vi "Aula do dia 03.02.vi"() -> (0 "Corrente Fase A":dynamicdata(graph), 1 "Tensão Fase A":dynamicdata(graph), 2 "Timestamp":dynamicdata(graph), 3 "Corrente Fase C":dynamicdata(graph), 4 "Tensão Fase C":dynamicdata(graph), 5 "Corrente Fase B":dynamicdata(graph), 6 "Tensão Fase B":dynamicdata(graph))   [LabVIEW 2020]
panel:
  out "Fase C":string[][](table)
  out "Fase B":string[][](table)
  out "Fase A":string[][](table)
  out "Timestamp":string[][](table)
  out "Gráfico de Ondas":dynamicdata(graph)
  out "All Data":string[][](table)
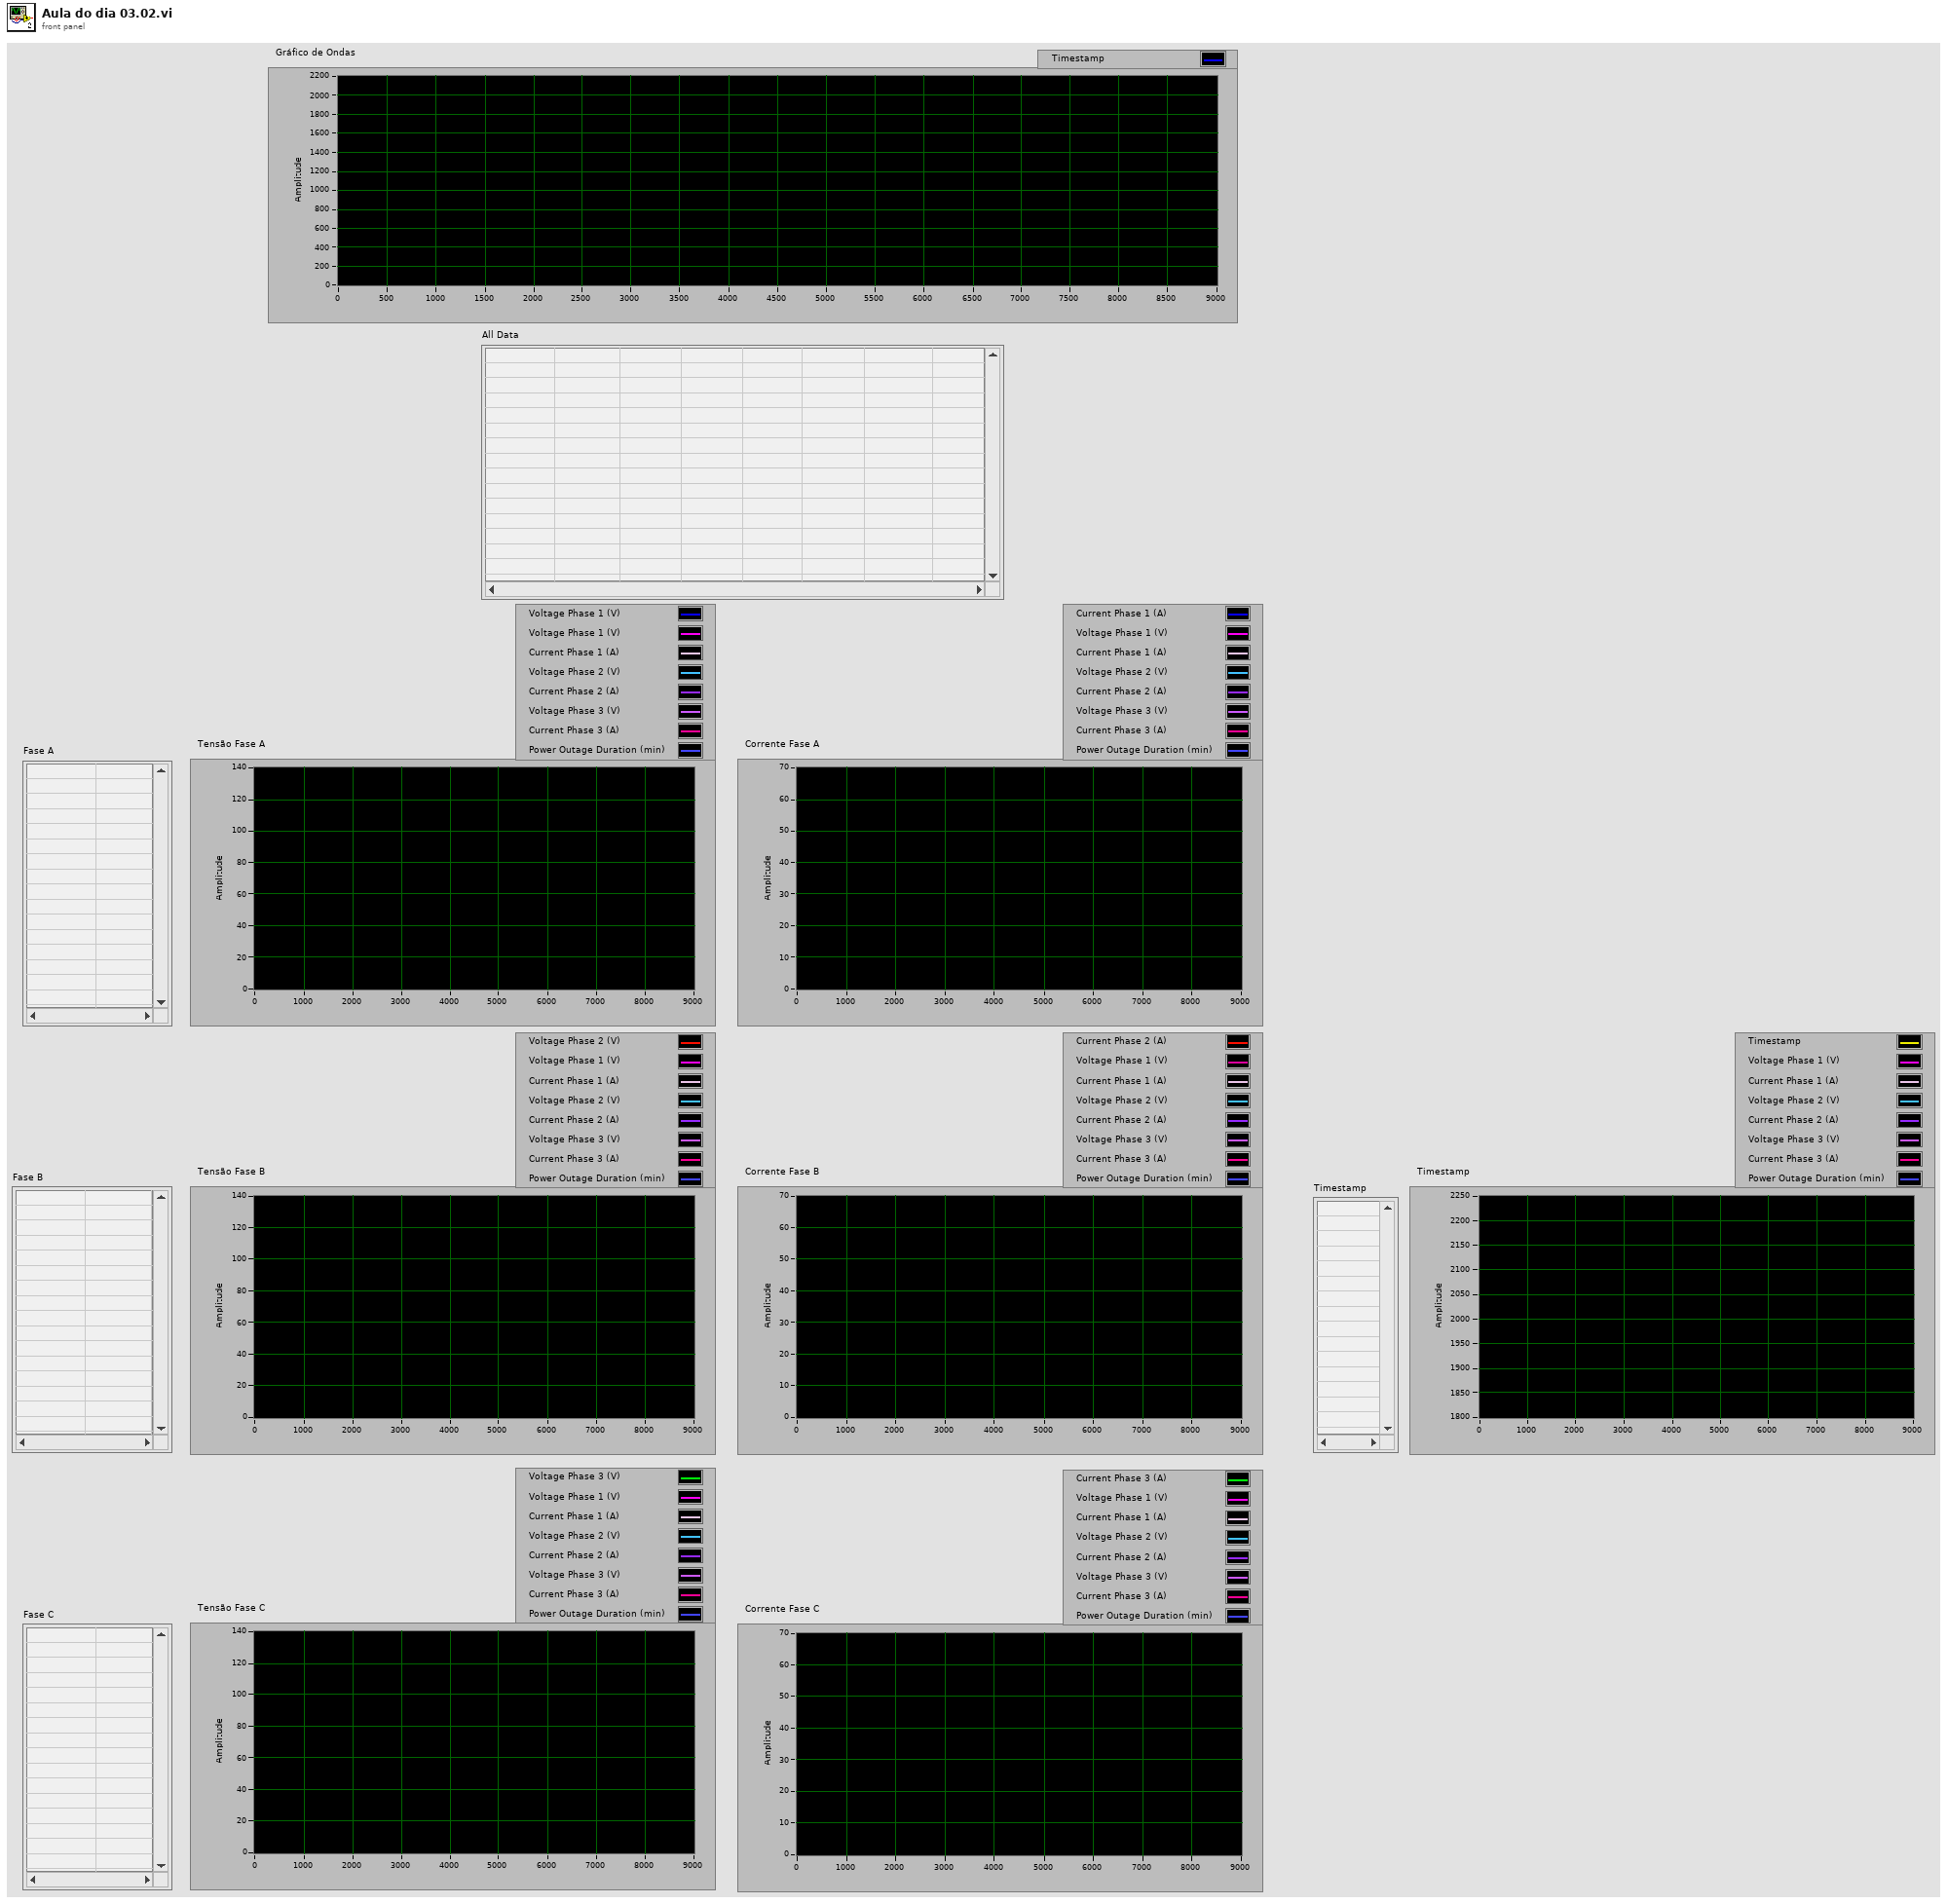
[diagram p1: front panel]
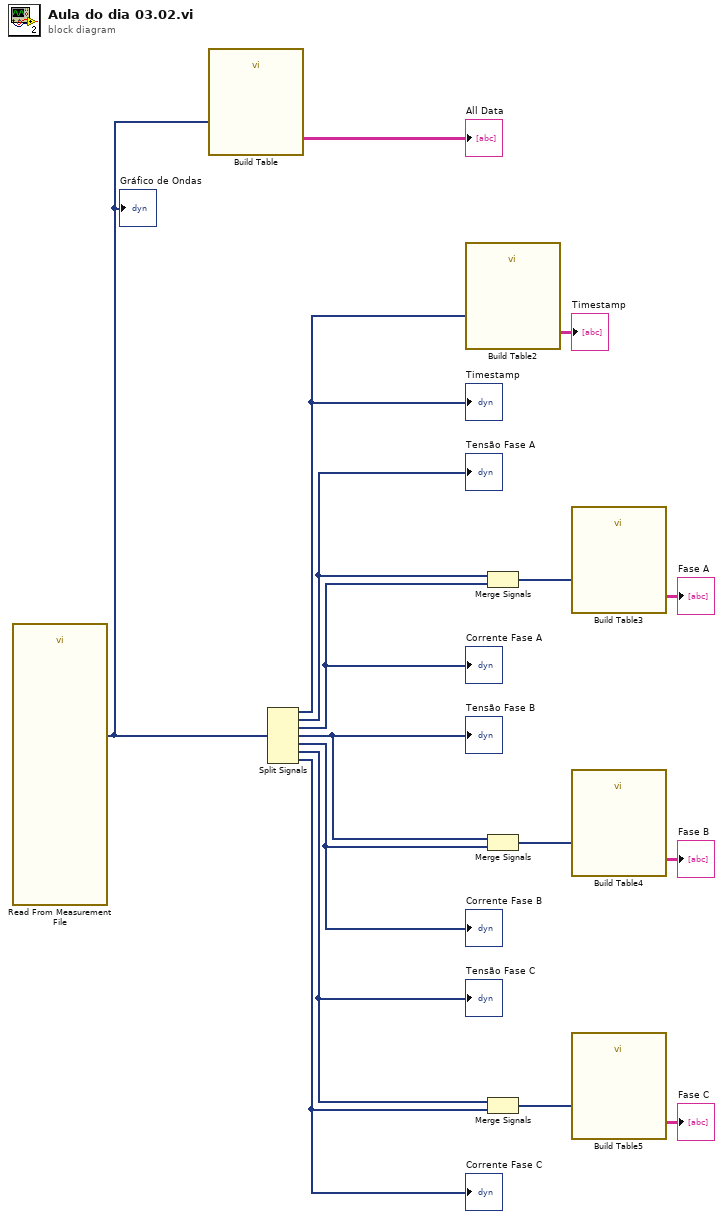
[diagram p0: block diagram]
diagram:
  n1 = call "Read From Measurement File"() -> ("Signals"=w15:dynamicdata)  [unwired: 6 in, 5 out]
  "Gráfico de Ondas" <- w15
  n2 = call "Build Table"("Signals"=w15) -> ("Table"=→"All Data":string[][])  [unwired: 4 in, 6 out]
  n3 = Split Signals(w15) -> (w12:dynamicdata, w11:dynamicdata, w9:dynamicdata, w7:dynamicdata, w6:dynamicdata, w2:dynamicdata, w1:dynamicdata)  [unwired: 7 in]
  "Timestamp" <- w12
  "Tensão Fase A" <- w11
  "Corrente Fase A" <- w9
  "Tensão Fase B" <- w7
  "Corrente Fase B" <- w6
  "Tensão Fase C" <- w2
  "Corrente Fase C" <- w1
  n4 = call "Build Table2"("Signals"=w12) -> ("Table"=→"Timestamp":string[][])  [unwired: 4 in, 6 out]
  n5 = Merge Signals(w11, w9) -> (w10:dynamicdata)
  n6 = Merge Signals(w7, w6) -> (w8:dynamicdata)
  n7 = Merge Signals(w2, w1) -> (w4:dynamicdata)
  n8 = call "Build Table3"("Signals"=w10) -> ("Table"=→"Fase A":string[][])  [unwired: 4 in, 6 out]
  n9 = call "Build Table4"("Signals"=w8) -> ("Table"=→"Fase B":string[][])  [unwired: 4 in, 6 out]
  n10 = call "Build Table5"("Signals"=w4) -> ("Table"=→"Fase C":string[][])  [unwired: 4 in, 6 out]
